vi "Show By Type.vi"(10 "Show":T2, 11 "Item's Property Type":T1(ring)) -> (3 "Show":bool)   [LabVIEW 2023]
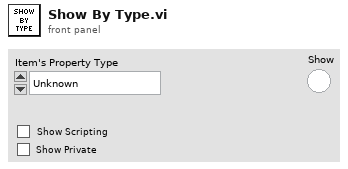
[diagram p1: front panel]
types:
  T1 = enum16{"Unknown", "Base", "Scripting", "Private", "Deprecated", "None", "Divider"}
  T2 = cluster{"Show Scripting":bool, "Show Private":bool}
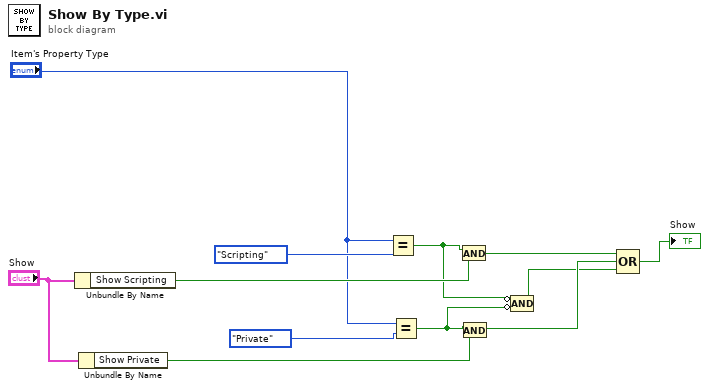
[diagram p0: block diagram]
diagram:
  n1 = Unbundle By Name("Show") -> ("Show Scripting"=w10:bool)
  n2 = Unbundle By Name("Show") -> ("Show Private"=w8:bool)
  n3 = Equal?(x="Item's Property Type", y=T1."Scripting" ("Property Type")) -> (x = y?=w3:bool)
  n4 = Equal?(x="Item's Property Type", y=T1."Private" ("Property Type")) -> (x = y?=w2:bool)
  n5 = And(x=w3, y=w10) -> (x .and. y?=w6:bool)
  n6 = And(x=w2, y=w8) -> (x .and. y?=w7:bool)
  n7 = Compound Arithmetic op=AND(invert w3, invert w2) -> (w1:bool)
  n8 = Compound Arithmetic op=OR(w6, w7, w1) -> (→"Show":bool)
